vi "TestFastExperimentCreate.vi"() -> ()   [LabVIEW 2017]
uses:
  Expose/Labview/Parameters/ExposeParameterBindingType.ctl
panel:
  out "id":string
  in  "TestMatrix":dbl[](array[numeric])
  out "ExpID":string
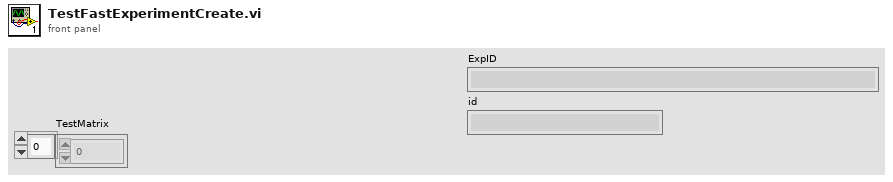
[diagram p1: front panel]
types:
  T1 = typedef "ExposeParameterBindingType.ctl" = enum16{"ToRemote", "FromRemote", "Bidrectional"}
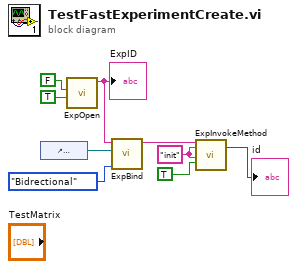
[diagram p0: block diagram]
diagram:
  w2 = "init" ("Method Name")
  n1 = control-ref of="TestMatrix"() -> (w7:refnum<vi>)
  n2 = call "ExpOpen.vi"("Do Expose Logging"=TRUE, "Requires Matlab Enviroment"=FALSE) -> ("ExpID"=w6:string)  [unwired: 7 in, 2 out]
  "ExpID" <- w6
  n3 = call "ExpBind.vi"("Binding Type"=ExposeParameterBindingType."Bidrectional", "Value"=w7, "ExpID"=w6) -> ("ExpID out"=w4:string)  [unwired: 7 in, 1 out]
  n4 = call "ExpInvokeMethod.vi"("ExpID"=w4, "Method Name"=w2, "Rsp. Type (or value to update)"=w2, "Require Response"=TRUE) -> ("Response"=→"id":variant)  [unwired: 13 in, 2 out]
